vi "CALC_SMO_POIN.vi"(0 "VISA IN":refnum<visa-resource-name>, 1 "Number of Points":i32, 5 "error in":errorcluster, 7 "Channel":i32) -> (14 "VISA Out":refnum<visa-resource-name>, 19 "error out":errorcluster)   [LabVIEW 2018, in "PNA-X.lvlib"]
doc: "CALCulate<cnum>:SMOothing:POINts <num> \n(Read-Write) Sets the number of adjacent data points to average. \nSee Critical Note \nParameters \n<cnum> Channel number of the measurement. There must be a selected measurement \non that channel. If unspecified, <cnum> is set to 1. \n<num> Number of points from 1 point to maximum of 25% of data points in the \nchannel. For example: if number of points in a data trace = 401, the maximum \nvalue for points = 100. The points value is always rounded to the closest odd \nnumber. \nExamples CALC:SMO:POIN 50 \ncalculate2:smoothing:points 21 \nQuery Syntax CALCulate<cnum>:SMOothing:POINts? \nReturn Type Numeric \nDefault 3"
uses:
  PNA-X.lvlib
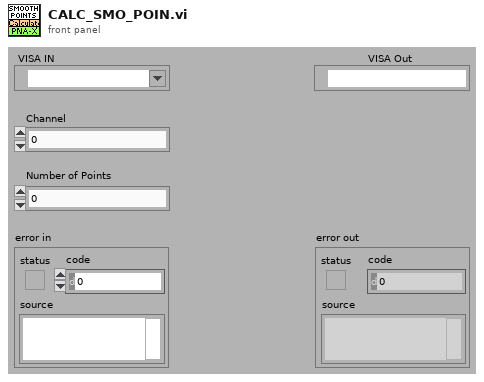
[diagram p1: front panel]
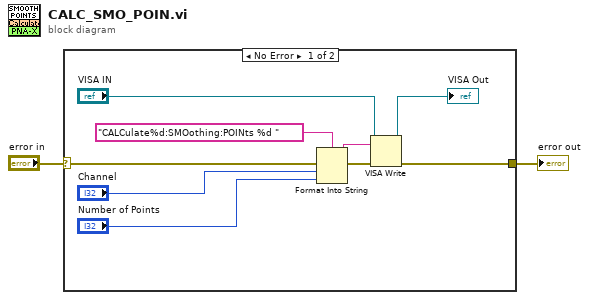
[diagram p0: block diagram]
diagram:
  n1 = case shown="No Error" "error in" {
    selector: "error in" -> [w11 w12]
    tunnel: [w6 w12] -> w1
    frame No Error {
      n2 = Format Into String(format string="CALCulate%d:SMOothing:POINts %d " ("Cmdline"), error in=w11, "Channel", "Number of Points") -> (resulting string=w9:string, error out=w10:errorcluster)  [unwired: 1 in]
      n3 = VISA Write(VISA resource name="VISA IN", write buffer=w9, error in (no error)=w10) -> (VISA resource name out=→"VISA Out":refnum<visa-resource-name>, error out=w6:errorcluster)  [unwired: 1 out]
    }
    frame Error {
    }
  }
  "error out" <- w1
